vi "SubVI RX Compute BER.vi"(4 "错误输入(无错误)":errorcluster, 6 "关键比特序列":u8[](array[numeric]), 7 "输入比特序列":u8[](array[numeric])) -> (0 "错误输出":errorcluster, 3 "误码率":dbl)   [LabVIEW 2015]
panel:
  # "计算误码率"
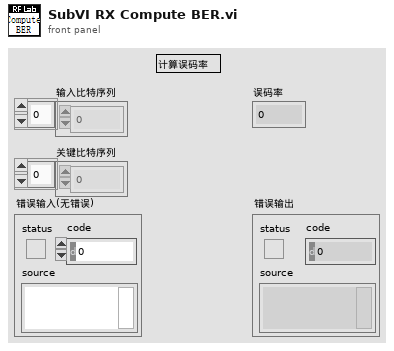
[diagram p1: front panel]
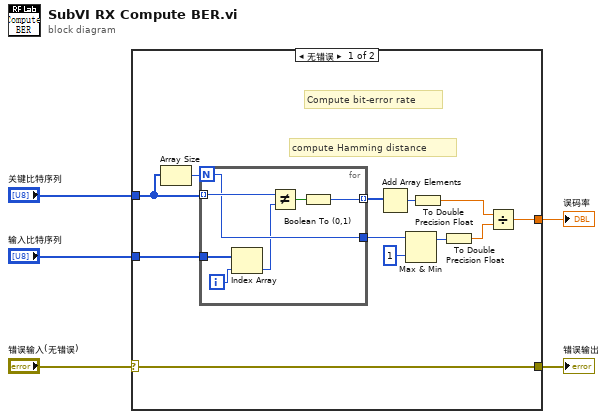
[diagram p0: block diagram]
diagram:
  n1 = case shown="无错误" "错误输入(无错误)" {
    selector: "错误输入(无错误)" -> [w9 w25]
    tunnel: [w9 w25] -> w4
    tunnel: "输入比特序列" -> [w8 _]
    tunnel: "关键比特序列" -> [w7 _]
    tunnel: [w6 _] -> w1
    frame No Error {
      # "Compute bit-error rate"
      # "compute Hamming distance"
      n2 = Array Size(array=w7) -> (size(s)=w17:i32)
      n3 = for {
        N: w17 -> [w21]
        tunnel: w7 -> [w23] mode=indexing
        tunnel: w8 -> [w20]
        tunnel: [w22] -> w11 mode=indexing
        tunnel: [w21] -> w10
        i -> [w19]
        n4 = Index Array(array=w20, index=w19) -> (element=w18:u8)
        n5 = Not Equal?(x=w23, y=w18) -> (x != y?=w24:bool)
        n6 = Boolean To (0,1)(Boolean=w24) -> (0, 1=w22:i16)
      }
      n7 = Add Array Elements(numeric array=w11) -> (sum=w12:i16)
      n8 = Max & Min(x=w10, y=1) -> (max(x,y)=w14:i32)  [unwired: 1 out]
      n9 = To Double Precision Float(number=w12) -> (double precision float=w15:dbl)
      n10 = To Double Precision Float(number=w14) -> (double precision float=w16:dbl)
      n11 = Divide(x=w15, y=w16) -> (x/y=w6:dbl)
    }
    frame Error {
    }
  }
  "错误输出" <- w4
  "误码率" <- w1
